vi "SCADA_Project (1).vi"() -> ()   [LabVIEW 2023]
uses:
  <vilib>/LabVIEW Interface for Arduino/LabVIEW Interface for Arduino.lvlib
panel:
  in  "VISA resource":refnum<visa-resource-name>
  in  "Smoke Value":dbl
  out "Smoke Output":dbl
  out "Voltage":dbl(knob) scale=0.0..5.0
  in  "Digital I/O Pin (0)":u8
  in  "Analog Input Pin (0)":u8
  in  "Stop":bool
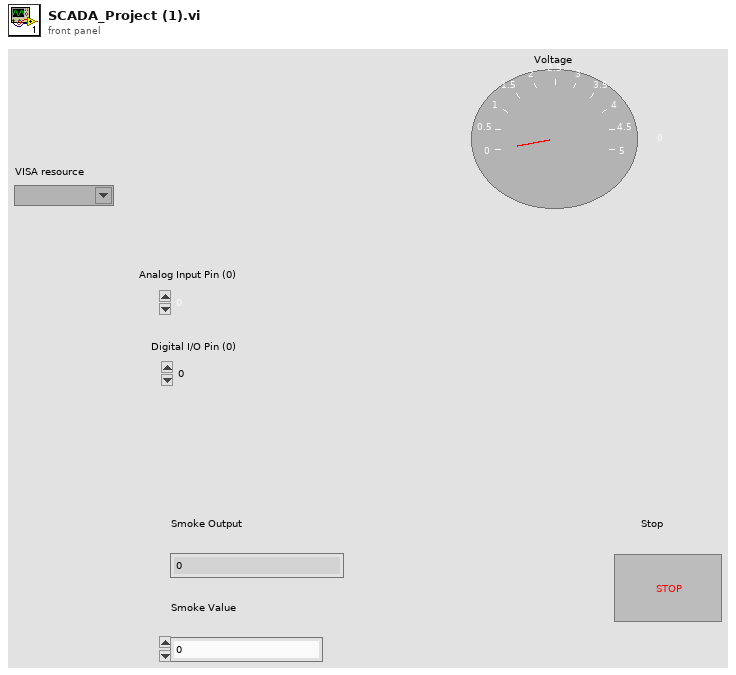
[diagram p1: front panel]
types:
  T1 = typedef "LabVIEW Interface for Arduino.lvlib/Arduino Resource.ctl" = cluster{"VISA resource":refnum<visa-resource-name>, "Board Type":T2, "Connection Type":enum8{"USB / Serial"}, "Bytes Per Packet (15)":u8}
  T2 = typedef "LabVIEW Interface for Arduino.lvlib/Board Type.ctl" = enum16{"Uno", "Dimuelanove w/Atmega 328", "Mega 2560"}
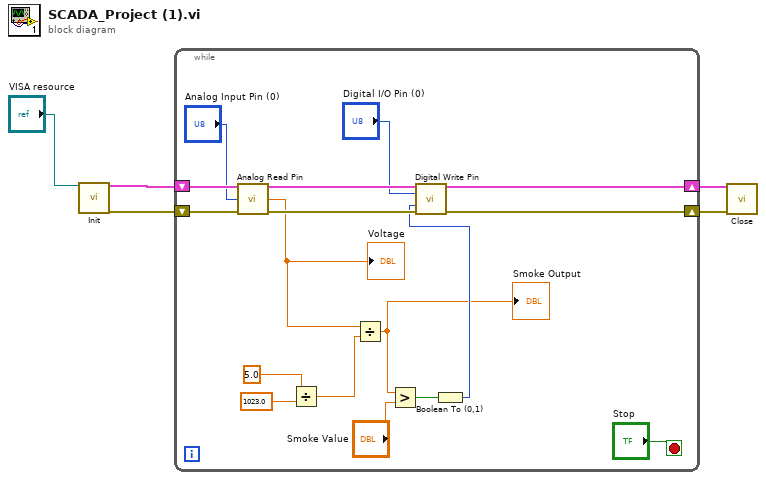
[diagram p0: block diagram]
diagram:
  n1 = call <vilib>:"Init.vi"("VISA resource"="VISA resource") -> ("Arduino Resource"=w5:T1, "error out"=w3:errorcluster)  [unwired: 17 in]
  n2 = while {
    shift-right: [w20] -> w4
    shift-left: w5 -> [w22]
    shift-right: [w17] -> w2
    shift-left: w3 -> [w19]
    stop <- "Stop" stop-if-true
    n3 = call <vilib>:"Analog Read Pin.vi"("Arduino Resource"=w22, "Analog Input Pin (0)"="Analog Input Pin (0)", "error in"=w19) -> ("Arduino Resource"=w21:T1, "Voltage"=w11:dbl, "error out"=w18:errorcluster)  [unwired: 10 in]
    "Voltage" <- w11
    n4 = Divide(x=5.0, y=1023.0) -> (x/y=w10:dbl)
    n5 = Divide(x=w11, y=w10) -> (x/y=w6:dbl)
    "Smoke Output" <- w6
    n6 = Greater?(x=w6, y="Smoke Value") -> (0:w8:bool)
    n7 = Boolean To (0,1)(Boolean=w8) -> (0, 1=w7:i16)
    n8 = call <vilib>:"Digital Write Pin.vi"("Arduino Resource"=w21, "Digital I/O Pin (0)"="Digital I/O Pin (0)", "Value (0)"=w7, "error in"=w18) -> ("Arduino Resource"=w20:T1, "error out"=w17:errorcluster)  [unwired: 10 in]
  }
  n9 = call <vilib>:"Close.vi"("Arduino Resource"=w4, "error in"=w2) -> ()  [unwired: 13 in, 1 out]
